vi "Motor_speed_controlling_with_PI_v7_closedloop.vi"() -> ()   [LabVIEW 2016]
doc: "This example demonstrates how to generate a PWM signal on a single channel using a LINX device."
uses:
  <vilib>/MakerHub/LINX/Public/Peripherals/Analog/Analog Read 1 Chan.vi
  <vilib>/MakerHub/LINX/Public/Peripherals/Digital/Digital Read 1 Chan.vi
  <vilib>/MakerHub/LINX/Public/Peripherals/PWM/PWM Set Duty Cycle 1 Chan.vi
  <vilib>/MakerHub/LINX/Public/Peripherals/Digital/Digital Write 1 Chan.vi
  <vilib>/MakerHub/LINX/Public/Peripherals/Analog/Analog Read N Chans.vi
  <vilib>/MakerHub/LINX/Public/Peripherals/Digital/Digital Read N Chans.vi
  <vilib>/MakerHub/LINX/Public/Peripherals/Digital/Digital Write N Chans.vi
  <vilib>/MakerHub/LINX/Private/Local IO/LinxAnalogRead.vi
  <vilib>/MakerHub/LINX/Public/Utilities/Check Channel.vi
  <vilib>/MakerHub/LINX/Private/Local IO/LinxDigitalRead.vi
  <vilib>/MakerHub/LINX/Private/Local IO/LinxDigitalWrite.vi
  <vilib>/MakerHub/LINX/Public/Utilities/Open Serial.vi
  <vilib>/MakerHub/LINX/Private/Utilties/Generate Error.vi
  <vilib>/addons/control/pid/pid.llb/PID (DBL).vi
  <vilib>/MakerHub/LINX/Public/Peripherals/PWM/PWM Set Duty Cycle N Chans.vi
  <vilib>/MakerHub/LINX/LMH-LINX.lvlib
  <vilib>/addons/control/pid/NI_PID_pid.lvlib
panel:
  out "output variable 3":dbl
  out "output variable 2":dbl
  out "output variable":dbl
  out "Loop Rate (Hz)":u32
  out "PWM Signal":dbl(graph)
  in  "Loop Delay(ms)":u32
  out "Motor Voltage":dbl(graph)
  out "PID Screen":cluster{"Motor Speed":dbl, "rpm":dbl}(graph)
  in  "Direction":bool
  out "Motor Speed(RPM)":cluster{dbl, dbl}(knob) scale=0.0..80.0
  in  "Encoder Input Pin":u8
  in  "PID gains":T1={"proportional gain (Kc)"=1.0, "integral time (Ti, min)"=0.01, "derivative time (Td, min)"=0.0} {"derivative time (Td, min)" format="%.3f"; "integral time (Ti, min)" format="%.3f"; "proportional gain (Kc)" format="%.3f"}
  in  "Motor Speed":dbl(knob) scale=0.0..80.0
  in  "PWM Output Pin":u8=3
  in  "Stop Button":bool
  in  "Serial Port":refnum<visa-resource-name>
  # "Direction"
  # "Motor Speed Control\n(RPM)"
  # "Motor Speed \n(RPM)"
  # "PID Settings"
  # "Device and Connection\nSettings"
  # "Forward"
  # "e"
  # "Back"
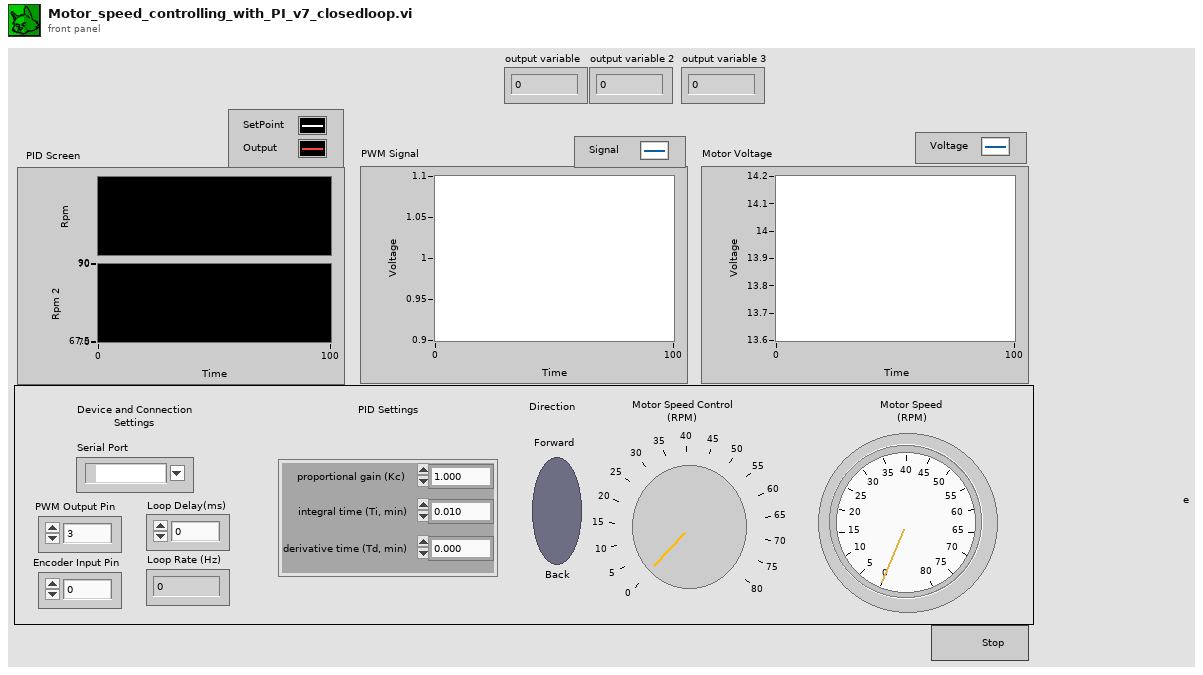
[diagram p1: front panel]
types:
  T1 = cluster{"proportional gain (Kc)":dbl, "integral time (Ti, min)":dbl, "derivative time (Td, min)":dbl}
  T2 = typedef "LMH-LINX.lvlib/LINX Ref.ctl" = cluster{"IO":T3, "Interface":T4, "LINX Device Config":T5}
  T3 = typedef "LMH-LINX.lvlib/Platform.ctl" = enum16{"Remote", "Local"}
  T4 = typedef "LMH-LINX.lvlib/Interface.ctl" = enum16{"Serial", "TCP"}
  T5 = typedef "LMH-LINX.lvlib/Device.lvlib/LINX Device Config.ctl" = cluster{"Interface":T4, "COM Port":refnum<visa-resource-name>, "TCP Configuration":T6, "Device Family":u8, "Device ID":u8, "Device Name":string, "TCP Ref":refnum<k5>, "Channels":T7}
  T6 = typedef "LMH-LINX.lvlib/Device.lvlib/TCP Config.ctl" = cluster{"IP Address":string, "Port":u16}
  T7 = typedef "LMH-LINX.lvlib/Channels.ctl" = cluster{"DI":u8[], "DO":u8[], "AI":u8[], "AO":u8[], "PWM":u8[], "QE":u8[], "UART":u8[], "I2C 2":u8[], "SPI":u8[], "CAN":u8[], "Servo":u8[], "AI Ref (V)":dbl, "AI Resolution (Bits)":u8, "AO Ref (V)":dbl, "AO Resolution (Bits)":u8}
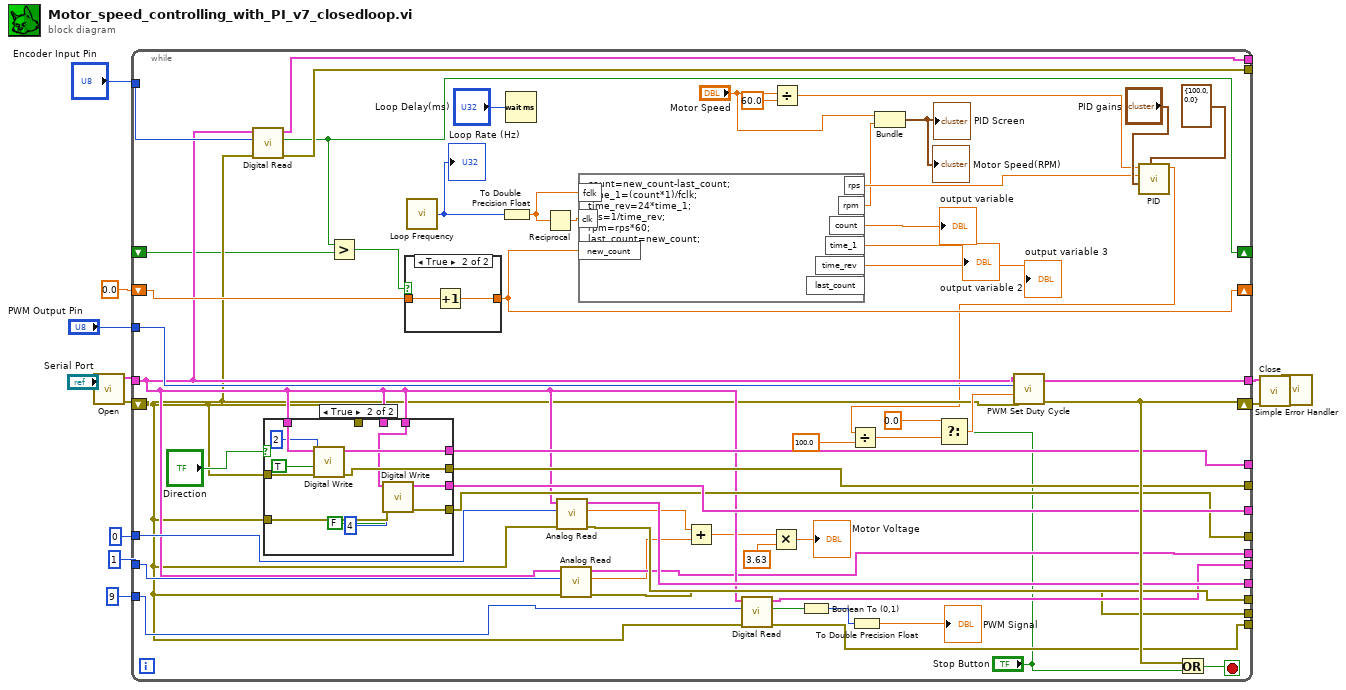
[diagram p0: block diagram]
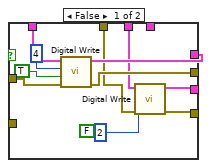
[diagram p3: hidden frame]
diagram:
  n1 = call-poly <vilib>:"Open.vi"("Serial Port"="Serial Port") -> ("Error Out"=w11:errorcluster, "LINX Resource"=w12:T2)  [unwired: 8 in, 1 out]
  n2 = while {
    tunnel: w12 -> [w38]
    tunnel: [w66] -> w10
    shift-right: [w68] -> w9
    shift-left: w11 -> [w37]
    tunnel: "PWM Output Pin" -> [w67]
    tunnel: "Encoder Input Pin" -> [w52]
    tunnel: [w51] -> _
    tunnel: [w50] -> _
    tunnel: [w60] -> _
    tunnel: [w59] -> _
    tunnel: [w56] -> _
    tunnel: [w55] -> _
    tunnel: [w54] -> _
    tunnel: [w53] -> _
    shift-right: [w18] -> _
    shift-left: _ -> [w17]
    shift-right: [w31] -> _
    shift-left: 0.0 -> [w48]
    tunnel: u8 0 ("Analog Channel") -> [w47]
    tunnel: [w46] -> _
    tunnel: [w45] -> _
    tunnel: u8 9 ("Analog Channel") -> [w42]
    tunnel: u8 1 ("Analog Channel") -> [w39]
    tunnel: [w36] -> _
    tunnel: [w35] -> _
    stop <- w69 stop-if-true
    n3 = call-poly <vilib>:"Digital Read.vi"("Error In"=w37, "DI Channel"=w52, "LINX Resource"=w38) -> ("Error Out"=w50:errorcluster, "DI Value"=w18:bool, "LINX Resource"=w51:T2)  [unwired: 6 in]
    n4 = case shown="True" "Direction" {
      tunnel: w38 -> [w84 w96]
      tunnel: w37 -> [w83 w95]
      tunnel: [w82 w93] -> w60
      tunnel: [w81 w92] -> w59
      tunnel: w38 -> [_ w90]
      tunnel: w37 -> [_ w89]
      tunnel: [w76 w88] -> w54
      tunnel: [w75 w87] -> w53
      tunnel: w38 -> [w78 _]
      tunnel: w37 -> [w77 _]
      frame False {
        n5 = call-poly <vilib>:"Digital Write.vi"("Error In"=w83, "Output Value"=TRUE, "DO Channel"=u8 4, "LINX Resource"=w84) -> ("Error Out"=w81:errorcluster, "LINX Resource"=w82:T2)  [unwired: 6 in]
        n6 = call-poly <vilib>:"Digital Write.vi"("Error In"=w77, "Output Value"=FALSE, "DO Channel"=u8 2, "LINX Resource"=w78) -> ("Error Out"=w75:errorcluster, "LINX Resource"=w76:T2)  [unwired: 6 in]
      }
      frame True {
        n7 = call-poly <vilib>:"Digital Write.vi"("Error In"=w95, "Output Value"=TRUE, "DO Channel"=u8 2, "LINX Resource"=w96) -> ("Error Out"=w92:errorcluster, "LINX Resource"=w93:T2)  [unwired: 6 in]
        n8 = call-poly <vilib>:"Digital Write.vi"("Error In"=w89, "Output Value"=FALSE, "DO Channel"=u8 4, "LINX Resource"=w90) -> ("Error Out"=w87:errorcluster, "LINX Resource"=w88:T2)  [unwired: 6 in]
      }
    }
    n9 = Greater?(x=w18, y=w17) -> (0:w16:bool)
    n10 = case shown="True" w16 {
      tunnel: w48 -> [w70 w72]
      tunnel: [w70 w71] -> w31
      frame False {
      }
      frame True {
        n11 = Increment(x=w72) -> (x+1=w71:dbl)
      }
    }
    n12 = call <vilib>:"Loop Frequency.vi"() -> ("Loop Rate (Hz)"=w30:u32)
    "Loop Rate (Hz)" <- w30
    n13 = To Double Precision Float(number=w30) -> (double precision float=w28:dbl)
    n14 = Wait (ms)(milliseconds to wait="Loop Delay(ms)") -> ()  [unwired: 1 out]
    n15 = Reciprocal(x=w28) -> (1/x=w27:dbl)
    n16 = call-poly <vilib>:"Analog Read.vi"("Error In"=w37, "Analog Channel"=w47, "LINX Resource"=w38) -> ("Error Out"=w55:errorcluster, "Voltage"=w34:dbl, "LINX Resource"=w56:T2)  [unwired: 5 in, 1 out]
    n17 = call-poly <vilib>:"Analog Read.vi"("Error In"=w37, "Analog Channel"=w39, "LINX Resource"=w38) -> ("Error Out"=w35:errorcluster, "Voltage"=w33:dbl, "LINX Resource"=w36:T2)  [unwired: 5 in, 1 out]
    n18 = formula code="count=new_count-last_count;\ntime_1=(count*1)/fclk;\ntime_rev=24*time_1;\nrps=1/time_rev;\nrpm=rps*60;\nlast_count=new_count;"("new_count"=w31, "fclk"=w28, "clk"=w27) -> ("time_1"=→"output variable 2":dbl, "rps"=w22:dbl, "count"=→"output variable":dbl, "time_rev"=→"output variable 3":dbl, "rpm"=w20:dbl)  [unwired: 1 out]
    n19 = Add(x=w34, y=w33) -> (x+y=w32:dbl)
    n20 = call-poly <vilib>:"Digital Read.vi"("Error In"=w37, "DI Channel"=w42, "LINX Resource"=w38) -> ("Error Out"=w45:errorcluster, "DI Value"=w29:bool, "LINX Resource"=w46:T2)  [unwired: 6 in]
    n21 = Multiply(x=w32, y=3.63) -> (x*y=→"Motor Voltage":dbl)
    n22 = Divide(x="Motor Speed", y=60.0) -> (x/y=w24:dbl)
    n23 = Boolean To (0,1)(Boolean=w29) -> (0, 1=w44:i16)
    n24 = To Double Precision Float(number=w44) -> (double precision float=→"PWM Signal":dbl)
    n25 = Bundle("Motor Speed"="Motor Speed", "rpm"=w20) -> (→"PID Screen" →"Motor Speed(RPM)":cluster{"Motor Speed":dbl, "rpm":dbl})  [unwired: 1 in]
    n26 = call-poly <vilib>:"PID.vi"("output range"=cluster{"output high":dbl, "output low":dbl} {"output high"=100.0, "output low"=0.0}, "PID gains"="PID gains", "process variable"=w22, "setpoint"=w24) -> ("output"=w19:dbl)  [unwired: 6 in, 1 out]
    n27 = Divide(x=w19, y=100.0) -> (x/y=w58:dbl)
    n28 = Select(t=0.0, s="Stop Button", f=w58) -> (s? t:f=w62:dbl)
    n29 = call-poly <vilib>:"PWM Set Duty Cycle.vi"("Error In"=w37, "Duty Cycle (0-1)"=w62, "PWM Channel"=w67, "LINX Resource"=w38) -> ("Error Out"=w68:errorcluster, "LINX Resource"=w66:T2)  [unwired: 6 in]
    n30 = Or(x=w68, y="Stop Button") -> (x .or. y?=w69:bool)
  }
  n31 = call <vilib>:"Close.vi"("Error In"=w9, "LINX Resource"=w10) -> ("Error Out"=w7:errorcluster)  [unwired: 9 in]
  n32 = call <vilib>:"Simple Error Handler.vi"("error in (no error)"=w7) -> ()  [unwired: 4 in, 5 out]
